vi "Selected 2 Pin Positions.vi"(10 "Selected":T2[](array[typedef])) -> (2 "Pin":T1[](array[typedef]))   [LabVIEW 2013]
uses:
  Selected Pin Positions.ctl
  lib/Data Access Objects/Metadata/Pin Positions.ctl
panel:
  # "Fixed"
  # "Platten"
  # "X"
  # "Z"
  # "X"
  # "Z"
  # "Y"
  # "Y"
  # "Fixed"
  # "Platten"
  # "X"
  # "Z"
  # "X"
  # "Z"
  # "Y"
  # "Y"
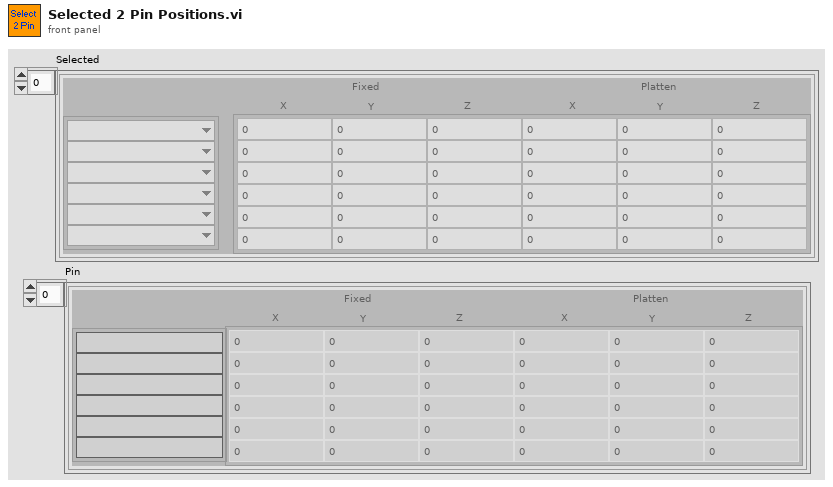
[diagram p1: front panel]
types:
  T1 = typedef "Pin Positions.ctl" = cluster{"Pin Positions":dbl[][], "Row Labels":string[]}
  T2 = typedef "Selected Pin Positions.ctl" = cluster{"Pin Positions":dbl[][], "Row Labels":u16[]}
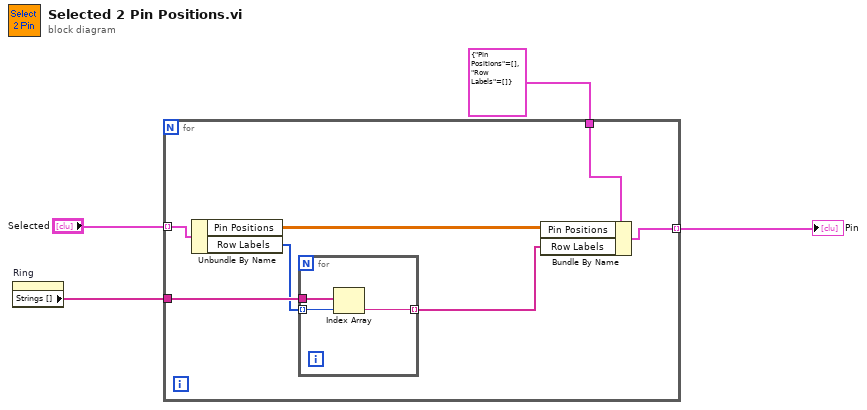
[diagram p0: block diagram]
diagram:
  n1 = property on="Ring" class="Ring (strict)"() -> ("Strings []"=w3:string[])  [unwired: 2 in, 2 out]
  n2 = for {
    tunnel: "Selected" -> [w11] mode=indexing
    tunnel: w3 -> [w10]
    tunnel: T1 {"Pin Positions"=[], "Row Labels"=[]} ("PinPositions") -> [w8]
    tunnel: [w5] -> w1 mode=indexing
    n3 = Unbundle By Name(w11) -> ("Pin Positions"=w7:dbl[][], "Row Labels"=w9:u16[])
    n4 = for {
      tunnel: w10 -> [w14]
      tunnel: w9 -> [w13] mode=indexing
      tunnel: [w12] -> w6 mode=indexing
      n5 = Index Array(array=w14, index=w13) -> (element=w12:string)
    }
    n6 = Bundle By Name(cluster=w8, "Pin Positions"=w7, "Row Labels"=w6) -> (w5:T1)
  }
  "Pin" <- w1
